vi "Disconnect All Channels.vi"(8 "error in (no error)":errorcluster, 11 "SLSC Switch in":refnum<class "SLSC Switch.lvclass">) -> (0 "error out":errorcluster, 3 "SLSC Switch out":refnum<class "SLSC Switch.lvclass">)   [LabVIEW 2016, in "SLSC Switch.lvlib" / "SLSC Switch.lvclass"]
doc: "Breaks all existing paths.\n\nIf the switch module cannot break all paths, a warning is returned. If an error in parameter describes an error that occurred before the call to this VI, SLSC-SWITCH still attempts to break all connections and returns the error information that was passed in from error in."
uses:
  SLSC Switch.lvclass
  Disconnect Channels (Multiple).vi
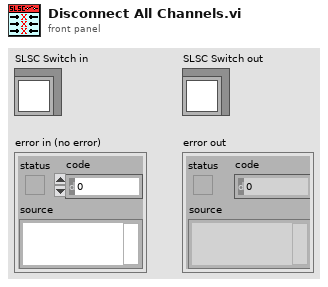
[diagram p1: front panel]
types:
  T1 = typedef "SLSC Switch.lvlib/SLSC Switch.lvclass/Connection.ctl" = cluster{"channel 1":string, "channel 2":string}
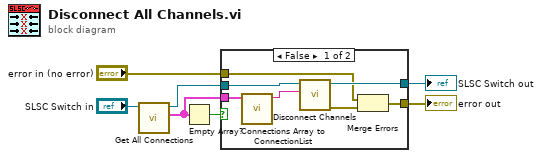
[diagram p0: block diagram]
diagram:
  n1 = call "Get All Connections.vi"("Route Manager in"="SLSC Switch in") -> ("connections"=w1:T1[], "Route Manager out"=w4:refnum<class "SLSC Switch.lvclass">)  [unwired: 9 in]
  n2 = Empty Array?(array=w1) -> (empty?=w2:bool)
  n3 = case shown="False" w2 {
    tunnel: [w14 w16] -> w6
    tunnel: [w13 w15] -> w3
    tunnel: w4 -> [w10 w15]
    tunnel: "error in (no error)" -> [w11 w16]
    tunnel: w1 -> [w9 _]
    frame False {
      n4 = call "Connections Array to ConnectionList.vi"("connections"=w9) -> ("connectionList"=w8:string)  [unwired: 10 in]
      n5 = call-poly "Disconnect Channels.vi"("disconnection list"=w8, "SLSC Switch in"=w10) -> ("error out"=w12:errorcluster, "SLSC Switch out"=w13:refnum<class "SLSC Switch.lvclass">)  [unwired: 8 in]
      n6 = Merge Errors(w11, w12) -> (w14:errorcluster)
    }
    frame True {
    }
  }
  "error out" <- w6
  "SLSC Switch out" <- w3
